vi "Pockels Cal-Message setup.vi"(8 "error in (no error)":errorcluster, 11 "State":T1) -> (0 "error out":errorcluster)   [LabVIEW 2013]
uses:
  Typedefs/Pockels cal wizard states.ctl
  Globals/gl_Calibration globals.vi
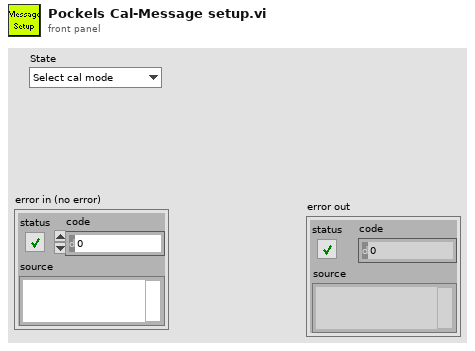
[diagram p1: front panel]
types:
  T1 = typedef "Pockels cal wizard states.ctl" = enum16{"Select cal mode", "Show instructions 1", "Select channel", "Show instructions 2", "Show instructions 3", "Confirm start", "Start calibration"}
  T2 = typedef "Pre-AOL Z wizard refs.ctl" = cluster{"VI's reference":refnum<vi>, "Calibration Mode":refnum<vi>, "Cal points":refnum<vi>, "Channel Selector":refnum<vi>, "Message":refnum<vi>, "Back":refnum<vi>, "Next":refnum<vi>, "Power meter AI":refnum<vi>, "2D Picture":refnum<vi>, "Note":refnum<vi>}
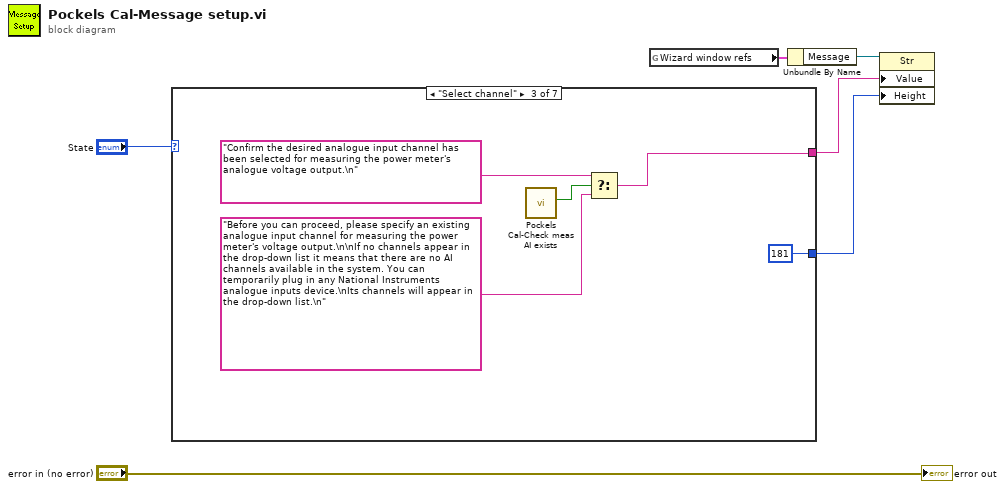
[diagram p0: block diagram]
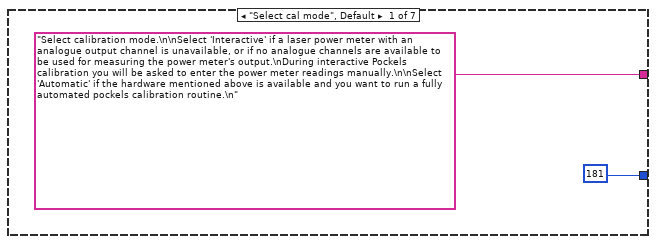
[diagram p2: hidden frame]
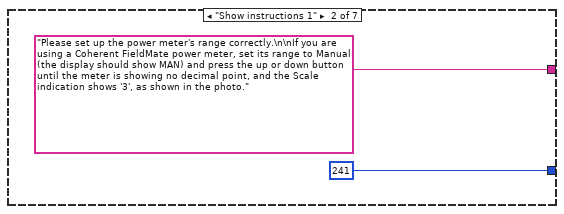
[diagram p3: hidden frame]
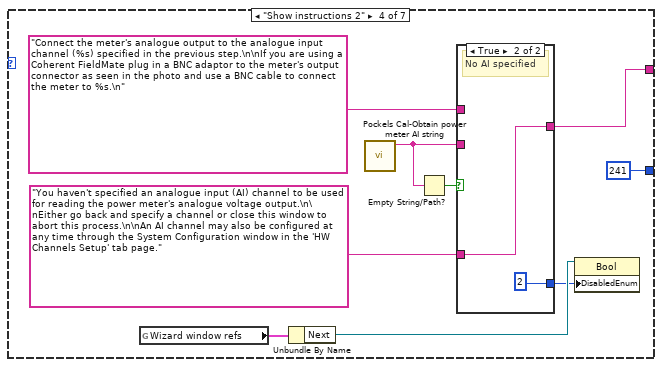
[diagram p4: hidden frame]
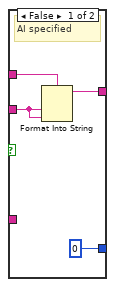
[diagram p5: hidden frame]
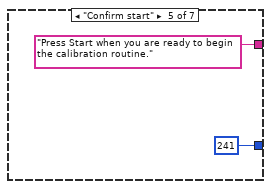
[diagram p6: hidden frame]
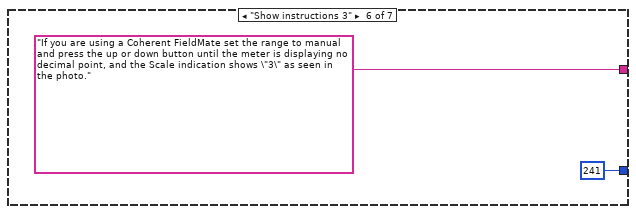
[diagram p7: hidden frame]
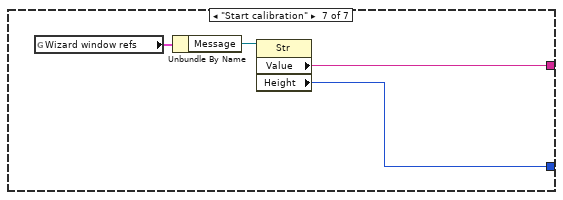
[diagram p8: hidden frame]
diagram:
  n1 = case shown="\"Select channel\"" "State" {
    tunnel: ["Select calibration mode.\n\nSelect 'Interactive' if a laser power meter with an analogue output channel is unavailable, or if no analogue channels are available to be used for measuring the power meter's output.\nDuring interactive Pockels calibration you will be asked to enter the power meter readings manually.\n\nSelect 'Automatic' if the hardware mentioned above is available and you want to run a fully automated pockels calibration routine.\n" ("Value") "Please set up the power meter's range correctly.\n\nIf you are using a Coherent FieldMate power meter, set its range to Manual (the display should show MAN) and press the up or down button until the meter is showing no decimal point, and the Scale indication shows '3', as shown in the photo." ("Value") w13 w23 "Press Start when you are ready to begin the calibration routine." ("Value") "If you are using a Coherent FieldMate set the range to manual and press the up or down button until the meter is displaying no decimal point, and the Scale indication shows \"3\" as seen in the photo." ("Value") w36] -> w2
    tunnel: [u32 181 ("Size:Height") u32 241 ("Size:Height") u32 181 ("Size:Height") u32 241 ("Size:Height") u32 241 ("Size:Height") u32 241 ("Size:Height") w35] -> w1
    frame "Select cal mode", Default {
    }
    frame "Show instructions 1" {
    }
    frame "Select channel" {
      n2 = call "Pockels Cal-Check meas AI exists.vi"() -> ("Power-meter meas. AI channel exists"=w14:bool)  [unwired: 9 in, 2 out]
      n3 = Select(t="Confirm the desired analogue input channel has been selected for measuring the power meter's analogue voltage output.\n" ("Value"), s=w14, f="Before you can proceed, please specify an existing analogue input channel for measuring the power meter's voltage output.\n\nIf no channels appear in the drop-down list it means that there are no AI channels available in the system. You can temporarily plug in any National Instruments analogue inputs device.\nIts channels will appear in the drop-down list.\n" ("Value")) -> (s? t:f=w13:string)
    }
    frame "Show instructions 2" {
      n4 = global read "gl_Calibration globals.vi" "Wizard window refs"() -> (w18:T2)
      n5 = Unbundle By Name(w18) -> ("Next"=w17:refnum<vi>)
      n6 = call "Pockels Cal-Obtain power meter AI string.vi"() -> ("Power meter AI (string)"=w22:string)  [unwired: 10 in, 1 out]
      n7 = Empty String/Path?(string/path=w22) -> (empty?=w21:bool)
      n8 = case shown="True" w21 {
        tunnel: "Connect the meter's analogue output to the analogue input channel (%s) specified in the previous step.\n\nIf you are using a Coherent FieldMate plug in a BNC adaptor to the meter's output connector as seen in the photo and use a BNC cable to connect the meter to %s.\n" ("Value") -> [w28 _]
        tunnel: [w27 w30] -> w23
        tunnel: w22 -> [w26 _]
        tunnel: "You haven't specified an analogue input (AI) channel to be used for reading the power meter's analogue voltage output.\n\nEither go back and specify a channel or close this window to abort this process.\n\nAn AI channel may also be configured at any time through the System Configuration window in the 'HW Channels Setup' tab page." ("Value") -> [_ w30]
        tunnel: [0 2] -> w16
        frame False {
          # "AI specified"
          n9 = Format Into String(format string=w28, w26, w26) -> (resulting string=w27:string)  [unwired: 2 in, 1 out]
        }
        frame True {
          # "No AI specified"
        }
      }
      n10 = property on="Property Node" class="Bool"(reference=w17, "DisabledEnum"=w16) -> ()  [unwired: 1 in, 2 out]
    }
    frame "Confirm start" {
    }
    frame "Show instructions 3" {
    }
    frame "Start calibration" {
      n11 = global read "gl_Calibration globals.vi" "Wizard window refs"() -> (w38:T2)
      n12 = Unbundle By Name(w38) -> ("Message"=w37:refnum<vi>)
      n13 = property on="Property Node" class="Str"(reference=w37) -> ("Value"=w36:string, "Height"=w35:u32)  [unwired: 1 in, 2 out]
    }
  }
  n14 = global read "gl_Calibration globals.vi" "Wizard window refs"() -> (w3:T2)
  n15 = Unbundle By Name(w3) -> ("Message"=w4:refnum<vi>)
  n16 = property on="Property Node" class="Str"(reference=w4, "Value"=w2, "Height"=w1) -> ()  [unwired: 1 in, 2 out]
  "error out" <- "error in (no error)"
